vi "Set Frequency.vi"(8 "error in (no error)":errorcluster, 10 "frequency(Hz)":dbl format="%_9p", 11 "VISA resource name":refnum<visa-resource-name>) -> (0 "error out":errorcluster)   [LabVIEW 2009]
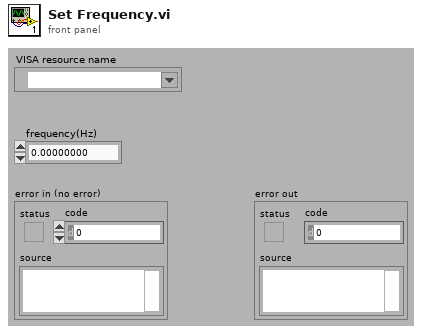
[diagram p1: front panel]
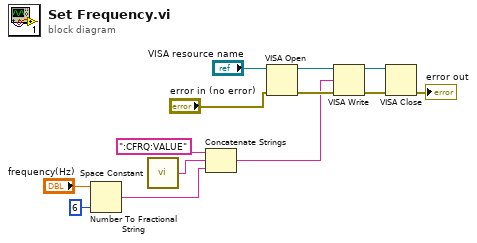
[diagram p0: block diagram]
diagram:
  n1 = Number To Fractional String(number="frequency(Hz)", precision (6)=i16 6) -> (F-format string=w5:string)  [unwired: 2 out]
  n2 = call <vilib>:"Space Constant.vi"() -> ("String"=w8:string)
  n3 = Concatenate Strings(":CFRQ:VALUE", w8, w5) -> (w4:string)
  n4 = VISA Open(error in (no error)="error in (no error)", VISA resource name="VISA resource name") -> (VISA resource name=w11:refnum<visa-resource-name>, error out=w10:errorcluster)  [unwired: 3 out]
  n5 = VISA Write(VISA resource name=w11, write buffer=w4, error in (no error)=w10) -> (VISA resource name out=w3:refnum<visa-resource-name>, error out=w2:errorcluster)  [unwired: 1 out]
  n6 = VISA Close(VISA resource name=w3, error in (no error)=w2) -> (error out=→"error out":errorcluster)
